vi "功率.vi"() -> ()   [LabVIEW 2022 SP3]
uses:
  <vilib>/Utility/file.llb/Read Delimited Spreadsheet (string).vi
panel:
  out "Array":string[][](array[string])
  in  "OK Button":bool
  out "累計功率":dbl
  out "即時功率":dbl
  out "即時電流":dbl
  out "即時電壓":dbl
  # "V"
  # "A"
  # "W"
  # "W"
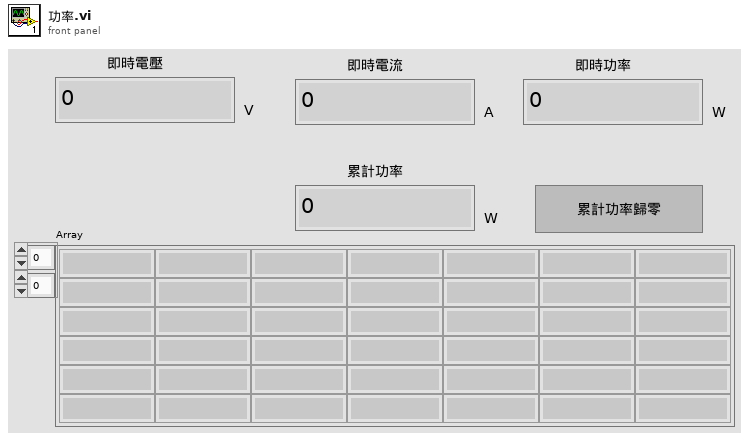
[diagram p1: front panel]
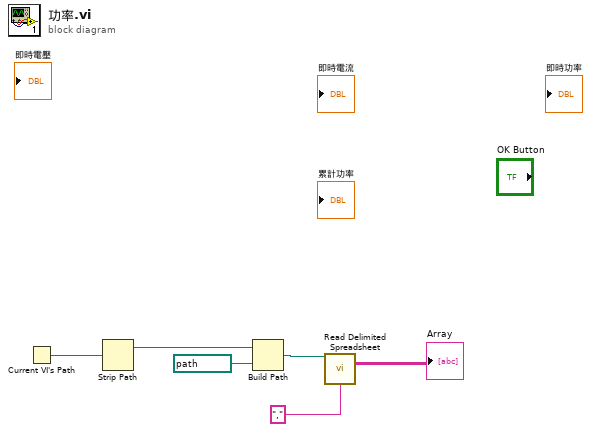
[diagram p0: block diagram]
diagram:
  n1 = Current VI's Path() -> (path=w2:path)
  n2 = Strip Path(path=w2) -> (stripped path=w3:path)  [unwired: 1 out]
  n3 = Build Path(base path=w3, name or relative path=path "功率.csv") -> (appended path=w5:path)
  n4 = call-poly <vilib>:"Read Delimited Spreadsheet.vi"("file path (dialog if empty)"=w5, "delimiter (\\t)"="," ("delimiter (\\t)")) -> ("all rows"=→"Array":string[][])  [unwired: 8 in, 5 out]
